vi "finduntracComport.vi"(3 "error IN":errorcluster) -> (8 "OUT COM":refnum<visa-resource-name>, 10 "error out":errorcluster)   [LabVIEW 2017]
uses:
  <vilib>/Instr/_visa.llb/VISA Find Search Mode.ctl
  <vilib>/Instr/_visa.llb/VISA Configure Serial Port (Instr).vi
panel:
  out "CONNECT OK":bool
  out "StateError":bool
  in  "termination char\n(0xA = '\\n' = LF)":u8=10 format="%.0x"
  out "find list":string[](array[string])
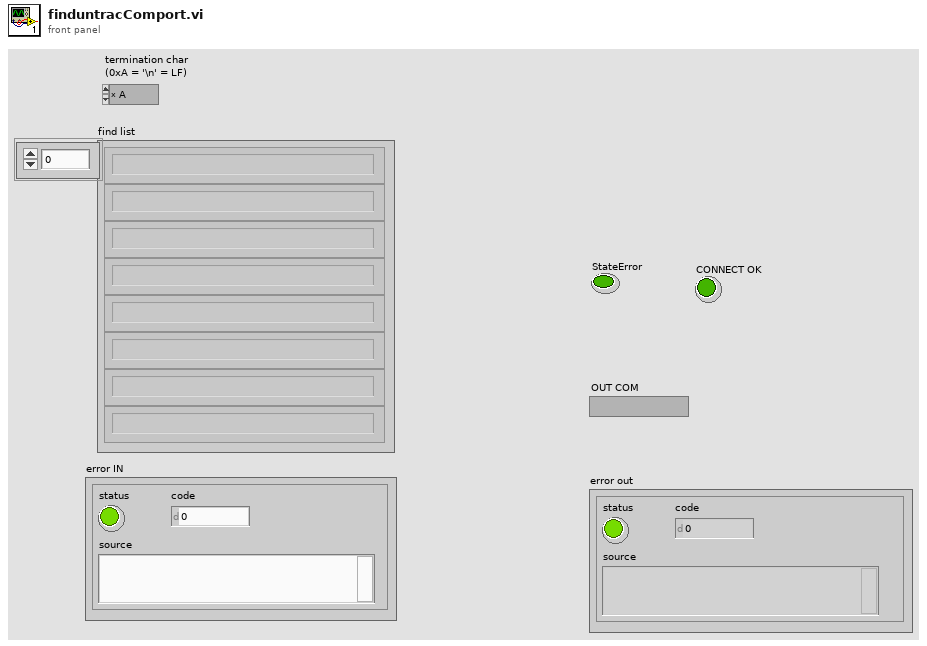
[diagram p1: front panel]
types:
  T1 = typedef "VISA Find Search Mode.ctl" = u32
  T2 = enum16{"InitCOM", "WriteCheck", "ReadCheck", "Comparedata", "End", "Stop"}
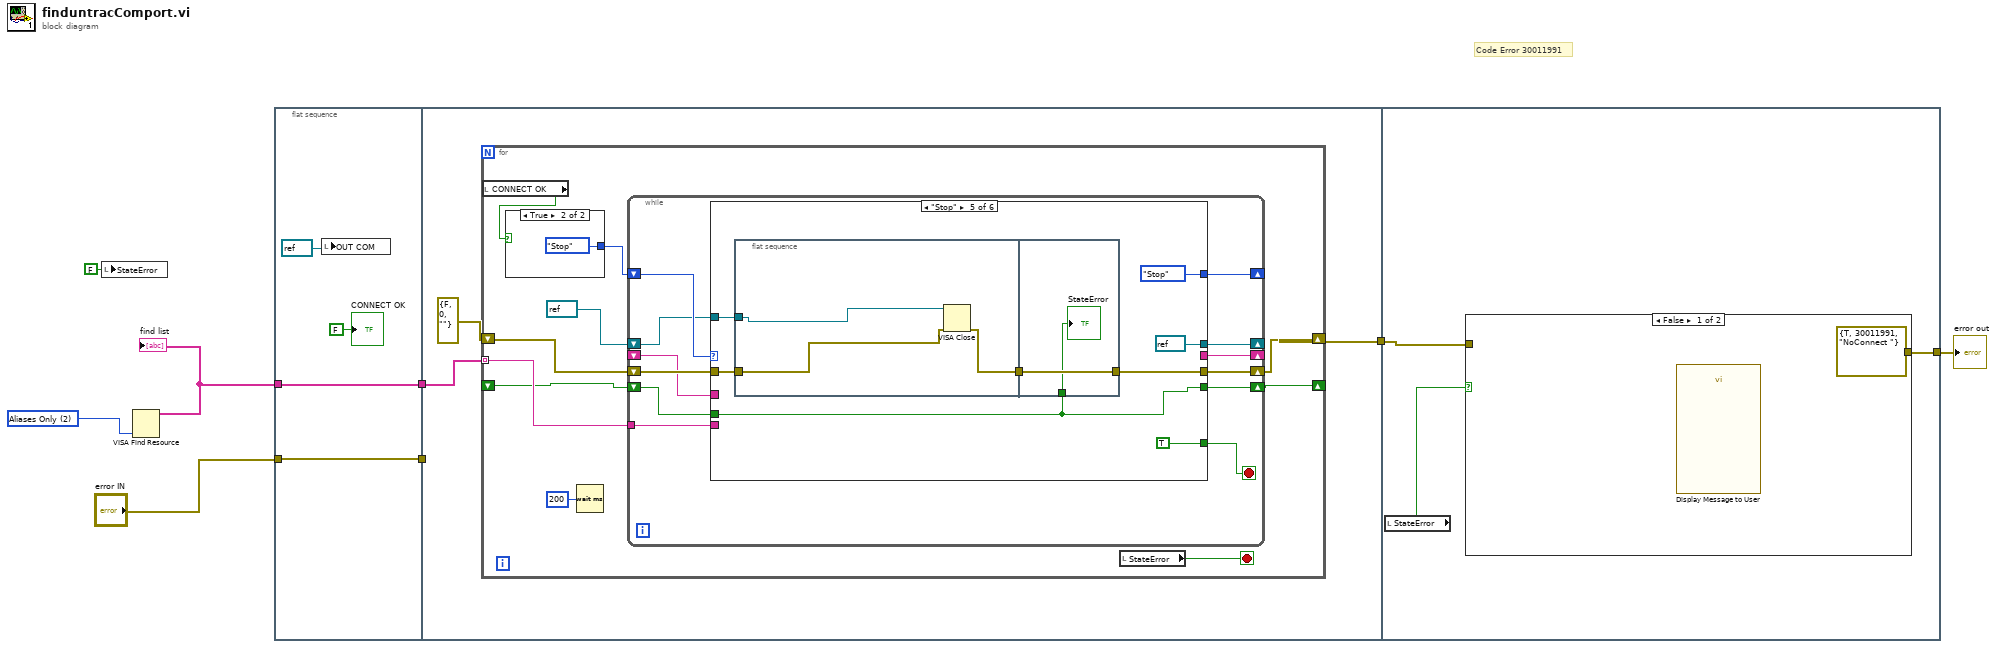
[diagram p0: block diagram]
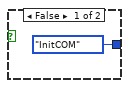
[diagram p2: hidden frame]
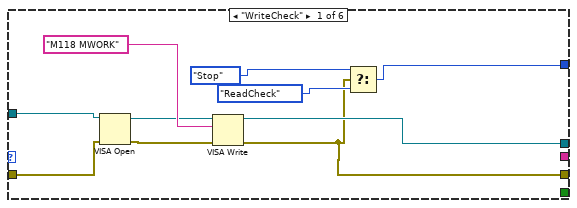
[diagram p3: hidden frame]
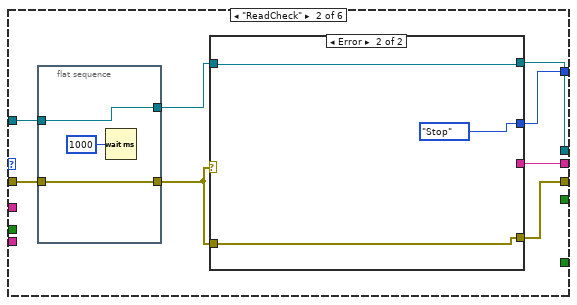
[diagram p4: hidden frame]
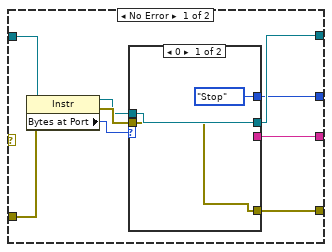
[diagram p5: hidden frame]
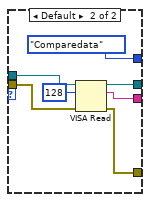
[diagram p6: hidden frame]
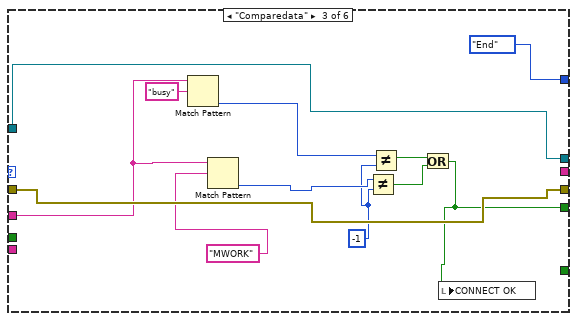
[diagram p7: hidden frame]
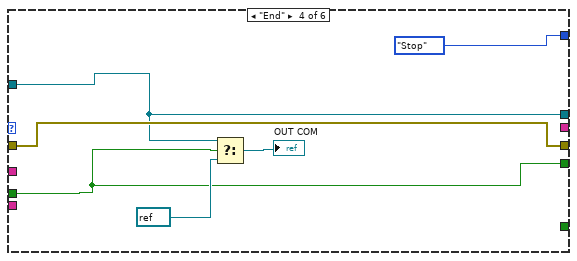
[diagram p8: hidden frame]
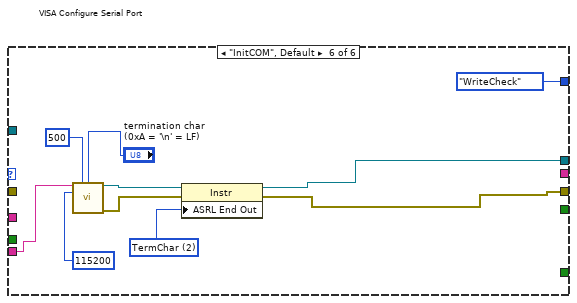
[diagram p9: hidden frame]
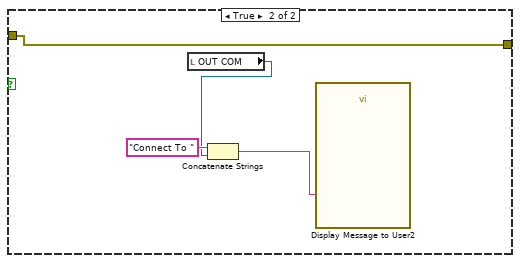
[diagram p10: hidden frame]
diagram:
  w8 = T1 2 items=["Canonical Names Only"=0, "Aliases Only"=2, "Include Matching Aliases"=3, "Include All Aliases"=4] ("Search Mode")
  # "Code Error 30011991"
  n1 = local write "StateError"(FALSE ("Boolean")) -> ()
  n2 = VISA Find Resource(10:w8) -> (3:w7:string[])  [unwired: 2 in, 2 out]
  "find list" <- w7
  n3 = flat-sequence {
    tunnel: "error IN" -> [w11]
    tunnel: w7 -> [w12]
    tunnel: [w12] -> w3
    tunnel: [w11] -> w2
    tunnel: [w14] -> w4
    tunnel: w3 -> [w15]
    tunnel: w2 -> [_]
    tunnel: w4 -> [w125]
    tunnel: [w124] -> w1
    frame #0 {
      n4 = local write "OUT COM"(refnum<visa-resource-name> refnum ("f")) -> ()
      "CONNECT OK" <- FALSE ("CONNECT OK")
    }
    frame #1 {
      n5 = for {
        tunnel: w15 -> [w23] mode=indexing
        shift-right: [w18] -> _
        shift-left: _ -> [w19]
        shift-right: [w25] -> w14
        shift-left: errorcluster {"status"=FALSE, "code"=0, "source"=""} ("error out") -> [w22]
        stop <- w20 stop-if-true
        n6 = local read "CONNECT OK"() -> (w17:bool)
        n7 = case shown="True" w17 {
          tunnel: [T2."InitCOM" ("State") T2."Stop" ("State")] -> w16
          frame False {
          }
          frame True {
          }
        }
        n8 = Wait (ms)(milliseconds to wait=u32 200) -> ()  [unwired: 1 out]
        n9 = while {
          shift-right: [w29] -> _
          shift-left: w16 -> [w39]
          shift-right: [w31] -> _
          shift-left: refnum<visa-resource-name> refnum ("VISA resource name out") -> [w38]
          shift-right: [w36] -> w25
          shift-left: w22 -> [w37]
          shift-right: [w35] -> _
          shift-left: _ -> [w34]
          shift-right: [w33] -> w18
          shift-left: w19 -> [w32]
          tunnel: w23 -> [w28]
          stop <- w30 stop-if-true
          n10 = case shown="\"Stop\"" w39 {
            tunnel: w38 -> [w46 w52 w94 w97 w105 _]
            tunnel: [w49 w56 w94 w97 refnum<visa-resource-name> refnum ("VISA resource name out") w115] -> w31
            tunnel: w37 -> [w47 w51 w91 w98 w106 _]
            tunnel: [w40 w57 w91 w98 w107 w114] -> w36
            tunnel: [_ w55 _ _ _ _] -> w35
            tunnel: w34 -> [_ _ w89 _ _ _]
            tunnel: [_ _ w85 w96 w102 _] -> w33
            tunnel: w32 -> [_ _ _ w96 w102 _]
            tunnel: [_ _ _ _ TRUE _] -> w30
            tunnel: [w43 w54 T2."End" ("State") T2."Stop" ("State") T2."Stop" ("State") T2."WriteCheck" ("State")] -> w29
            tunnel: w28 -> [_ _ _ _ _ w116]
            frame "WriteCheck" {
              n11 = VISA Open(error in (no error)=w47, VISA resource name=w46) -> (VISA resource name=w44:refnum<visa-resource-name>, error out=w45:errorcluster)  [unwired: 3 in]
              n12 = VISA Write(VISA resource name=w44, write buffer="M118 MWORK" ("string"), error in (no error)=w45) -> (VISA resource name out=w49:refnum<visa-resource-name>, error out=w40:errorcluster)  [unwired: 1 out]
              n13 = Select(t=T2."Stop" ("f"), s=w40, f=T2."ReadCheck" ("State")) -> (s? t:f=w43:T2)
            }
            frame "ReadCheck" {
              n14 = flat-sequence {
                tunnel: [w60] -> w53
                tunnel: w52 -> [w60]
                tunnel: [w59] -> w50
                tunnel: w51 -> [w59]
                frame #0 {
                  n15 = Wait (ms)(milliseconds to wait=u32 1000) -> ()  [unwired: 1 out]
                }
              }
              n16 = case shown="Error" w50 {
                tunnel: [w64 w81] -> w57
                tunnel: w50 -> [w68 w81]
                tunnel: w53 -> [w69 w82]
                tunnel: [w65 w82] -> w56
                tunnel: [w63 _] -> w55
                tunnel: [w62 T2."Stop" ("State")] -> w54
                frame No Error {
                  n17 = property class="Instr"(reference=w69, error in=w68) -> (reference out=w66:refnum<visa-resource-name>, error out=w67:errorcluster, "Bytes at Port"=w61:u32)
                  n18 = case shown="0" w61 {
                    tunnel: w67 -> [w70 w79]
                    tunnel: w66 -> [w71 w78]
                    tunnel: [w71 w77] -> w65
                    tunnel: [w70 w76] -> w64
                    tunnel: [_ w75] -> w63
                    tunnel: [T2."Stop" ("State") T2."Comparedata" ("State")] -> w62
                    frame 0 {
                    }
                    frame Default {
                      n19 = VISA Read(VISA resource name=w78, byte count=u32 128, error in (no error)=w79) -> (VISA resource name out=w77:refnum<visa-resource-name>, read buffer=w75:string, error out=w76:errorcluster)  [unwired: 1 out]
                    }
                  }
                }
                frame Error {
                }
              }
            }
            frame "Comparedata" {
              w86 = -1 ("y")
              n20 = Match Pattern(string=w89, regular expression="busy") -> (offset past match=w87:i32)  [unwired: 1 in, 3 out]
              n21 = Match Pattern(string=w89, regular expression="MWORK" ("search string")) -> (offset past match=w92:i32)  [unwired: 1 in, 3 out]
              n22 = Not Equal?(x=w92, y=w86) -> (x != y?=w83:bool)
              n23 = Not Equal?(x=w87, y=w86) -> (x != y?=w84:bool)
              n24 = Or(x=w84, y=w83) -> (x .or. y?=w85:bool)
              n25 = local write "CONNECT OK"(w85) -> ()
            }
            frame "End" {
              n26 = Select(t=w97, s=w96, f=refnum<visa-resource-name> refnum) -> (s? t:f=→"OUT COM":refnum<visa-resource-name>)
            }
            frame "Stop" {
              n27 = flat-sequence {
                tunnel: w106 -> [w109]
                tunnel: w105 -> [w110]
                tunnel: [w111] -> w103
                tunnel: [w113] -> w107
                tunnel: w103 -> [w113]
                tunnel: w102 -> [w112]
                frame #0 {
                  n28 = VISA Close(VISA resource name=w110, error in (no error)=w109) -> (error out=w111:errorcluster)
                }
                frame #1 {
                  "StateError" <- w112
                }
              }
            }
            frame "InitCOM", Default {
              w122 = u16 2 items=["None", "Last Bit", "TermChar", "Break"] ("Serial Settings:End Mode for Writes")
              n29 = call-poly "VISA Configure Serial Port"("VISA resource name"=w116, "timeout (10sec)"=u32 500, "termination char\n(0xA = '\\n' = LF)"="termination char\n(0xA = '\\n' = LF)", "baud rate (9600)"=u32 115200) -> ("VISA resource name out"=w120:refnum<visa-resource-name>, "error out"=w121:errorcluster)  [unwired: 10 in]
              n30 = property class="Instr"(reference=w120, error in=w121, "ASRL End Out"=w122) -> (reference out=w115:refnum<visa-resource-name>, error out=w114:errorcluster)
            }
          }
        }
        n31 = local read "StateError"() -> (w20:bool)
      }
    }
    frame #2 {
      n32 = local read "StateError"() -> (w126:bool)
      n33 = case shown="False" w126 {
        tunnel: w125 -> [_ w128]
        tunnel: [errorcluster {"status"=TRUE, "code"=30011991, "source"="NoConnect "} ("error out") w128] -> w124
        frame False {
          n34 = call "Display Message to User"() -> ()  [unwired: 10 in, 2 out]
        }
        frame True {
          n35 = local read "OUT COM"() -> (w129:refnum<visa-resource-name>)
          n36 = Concatenate Strings("Connect To " ("string"), w129) -> (w131:string)
          n37 = call "Display Message to User2"("Message"=w131) -> ()  [unwired: 9 in, 2 out]
        }
      }
    }
  }
  "error out" <- w1
